vi "Main_ch.vi"() -> ()   [LabVIEW 2020]
uses:
  <vilib>/Utility/error.llb/DialogType.ctl
  <vilib>/DAQmx/read.llb/DAQmx Read (Analog 1D Wfm NChan NSamp).vi
  <extravilib>/ChannelInstances/Tag-bool/Read With Abort.vi
  <extravilib>/ChannelInstances/Tag-bool/Write With Abort.vi
  <vilib>/ULx/Create Channel.llb/ULx Create Channel (AI-Voltage-Basic).vi
  <vilib>/ULx/Timing.llb/ULx Timing (Sample Clock).vi
  <vilib>/DAQmx/create/channels.llb/DAQmx Create Channel (AI-Acceleration-Accelerometer).vi
  <vilib>/DAQmx/configure/timing.llb/DAQmx Timing (Sample Clock).vi
  <vilib>/DAQmx/configure/trigger.llb/DAQmx Start Trigger (Digital Edge).vi
  <vilib>/DAQmx/configure/trigger.llb/DAQmx Start Trigger (Time).vi
  <vilib>/DAQmx/configure/trigger.llb/DAQmx Start Trigger (Analog Edge).vi
  <extravilib>/ChannelInstances/Tag-bool/Instantiate.vi
  <extravilib>/ChannelInstances/Tag-bool/EndpointRead.vi
  <vilib>/ULx/Read.llb/ULx Read (Analog Wfm 1Chan NSamp).vi
  <vilib>/Waveform/DWDTOps.llb/DWDT Digital to Binary U16.vi
  <vilib>/ULx/Read.llb/ULx Read (Analog 1D Wfm NChan NSamp).vi
  <vilib>/DAQmx/miscellaneous.llb/DAQmx Fill In Error Info.vi
  <extravilib>/ChannelInstances/Tag-bool/Endpoint.vi
  <extravilib>/ChannelInstances/Tag-bool.lvlib
  <resource>/objmgr/daqmx.rc
panel:
  out "Power Graph":waveform(dbl)(graph)
  out "Tach Graph":digitalwaveform[](graph)
  out "Torque Graph":waveform(dbl)(graph)
  in  "Trigger Type":T1(tab)
  in  "Digital Start Trigger Edge":i32(ring)=10280 caption="Edge" items=["Rising"=10280, "Falling"=10171]
  in  "Digital Start Trigger Source":tag="/Dev1/PFI0" caption="Source"
  in  "Digital Pause Trigger Pause When":i32(ring)=10192 caption="Pause When" items=["High"=10192, "Low"=10214]
  in  "Digital Pause Trigger Source":tag="/Dev1/PFI0" caption="Source"
  in  "Analog Start Trigger Level":dbl caption="Level" format="%0.2f"
  in  "Analog Start Trigger Hysteresis":dbl caption="Hysteresis" format="%.2f"
  in  "Analog Start Trigger Slope":i32(ring)=10280 caption="Slope" items=["Rising"=10280, "Falling"=10171]
  in  "Analog Start Trigger Source":string="APFI0" caption="Source"
  in  "Analog Pause Trigger Source":string="APFI0" caption="Source"
  in  "Analog Pause Trigger Pause When":i32(ring)=10093 caption="Pause When" items=["Above Level"=10093, "Below Level"=10107]
  in  "Analog Pause Trigger Level":dbl caption="Level" format="%.2f"
  in  "When":timestamp
  in  "Select Time\nManually":bool
  out "Accel Graph":waveform(dbl)[](graph)
  out "Actual Sample Rate":dbl=1000.0 format="%0.2f"
  out "Mic Graph":dynamicdata(graph)
  out "Load Cell Graph":waveform(dbl)[](graph)
  in  "stop":bool
  # "To enable triggers, select a tab above, and configure the settings.\n\nNot all hardware supports all trigger types. Refer to your device documentation for more information."
  # "This trigger type is not supported in continuous sample timing. \n\nRefer to your device documentation for more information on which triggers are supported."
  # "This trigger type is not supported in continuous sample timing. \n\nRefer to your device documentation for more information on which triggers are supported."
  # "If time is not manually set, task will begin after 10 seconds"
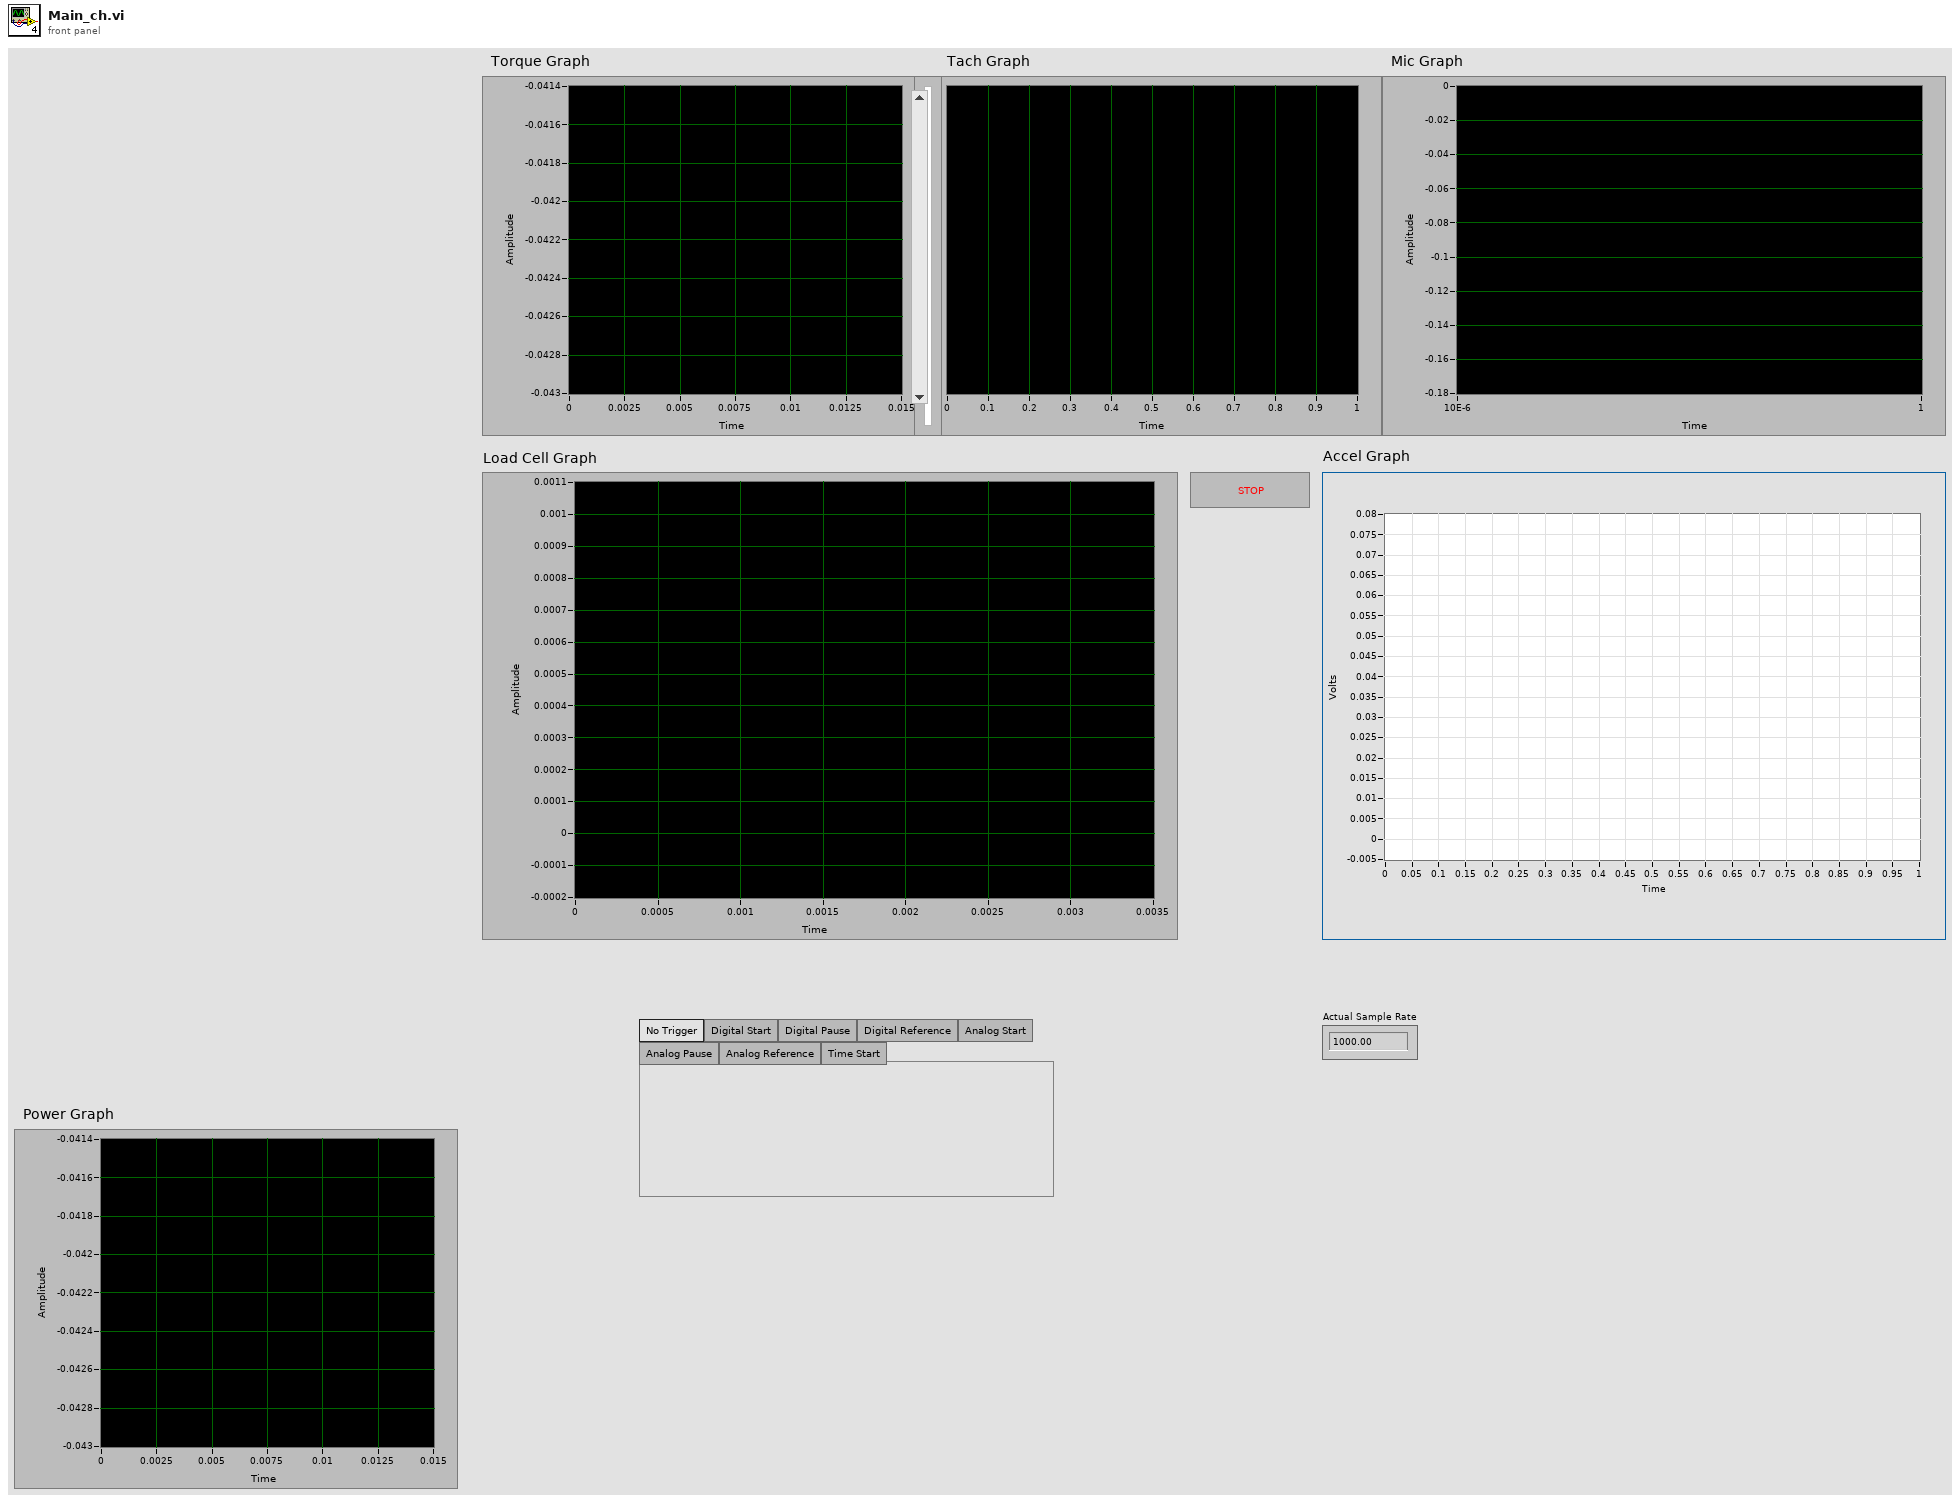
[diagram p1: front panel]
types:
  T1 = enum32{"No Trigger", "Digital Start", "Digital Pause", "Digital Reference", "Analog Start", "Analog Pause", "Analog Reference", "Time Start"}
  T2 = typedef "DialogType.ctl" = u16
  T3 = typedef "Tag-bool.lvlib/))Channel.ctl" = refnum<queue>
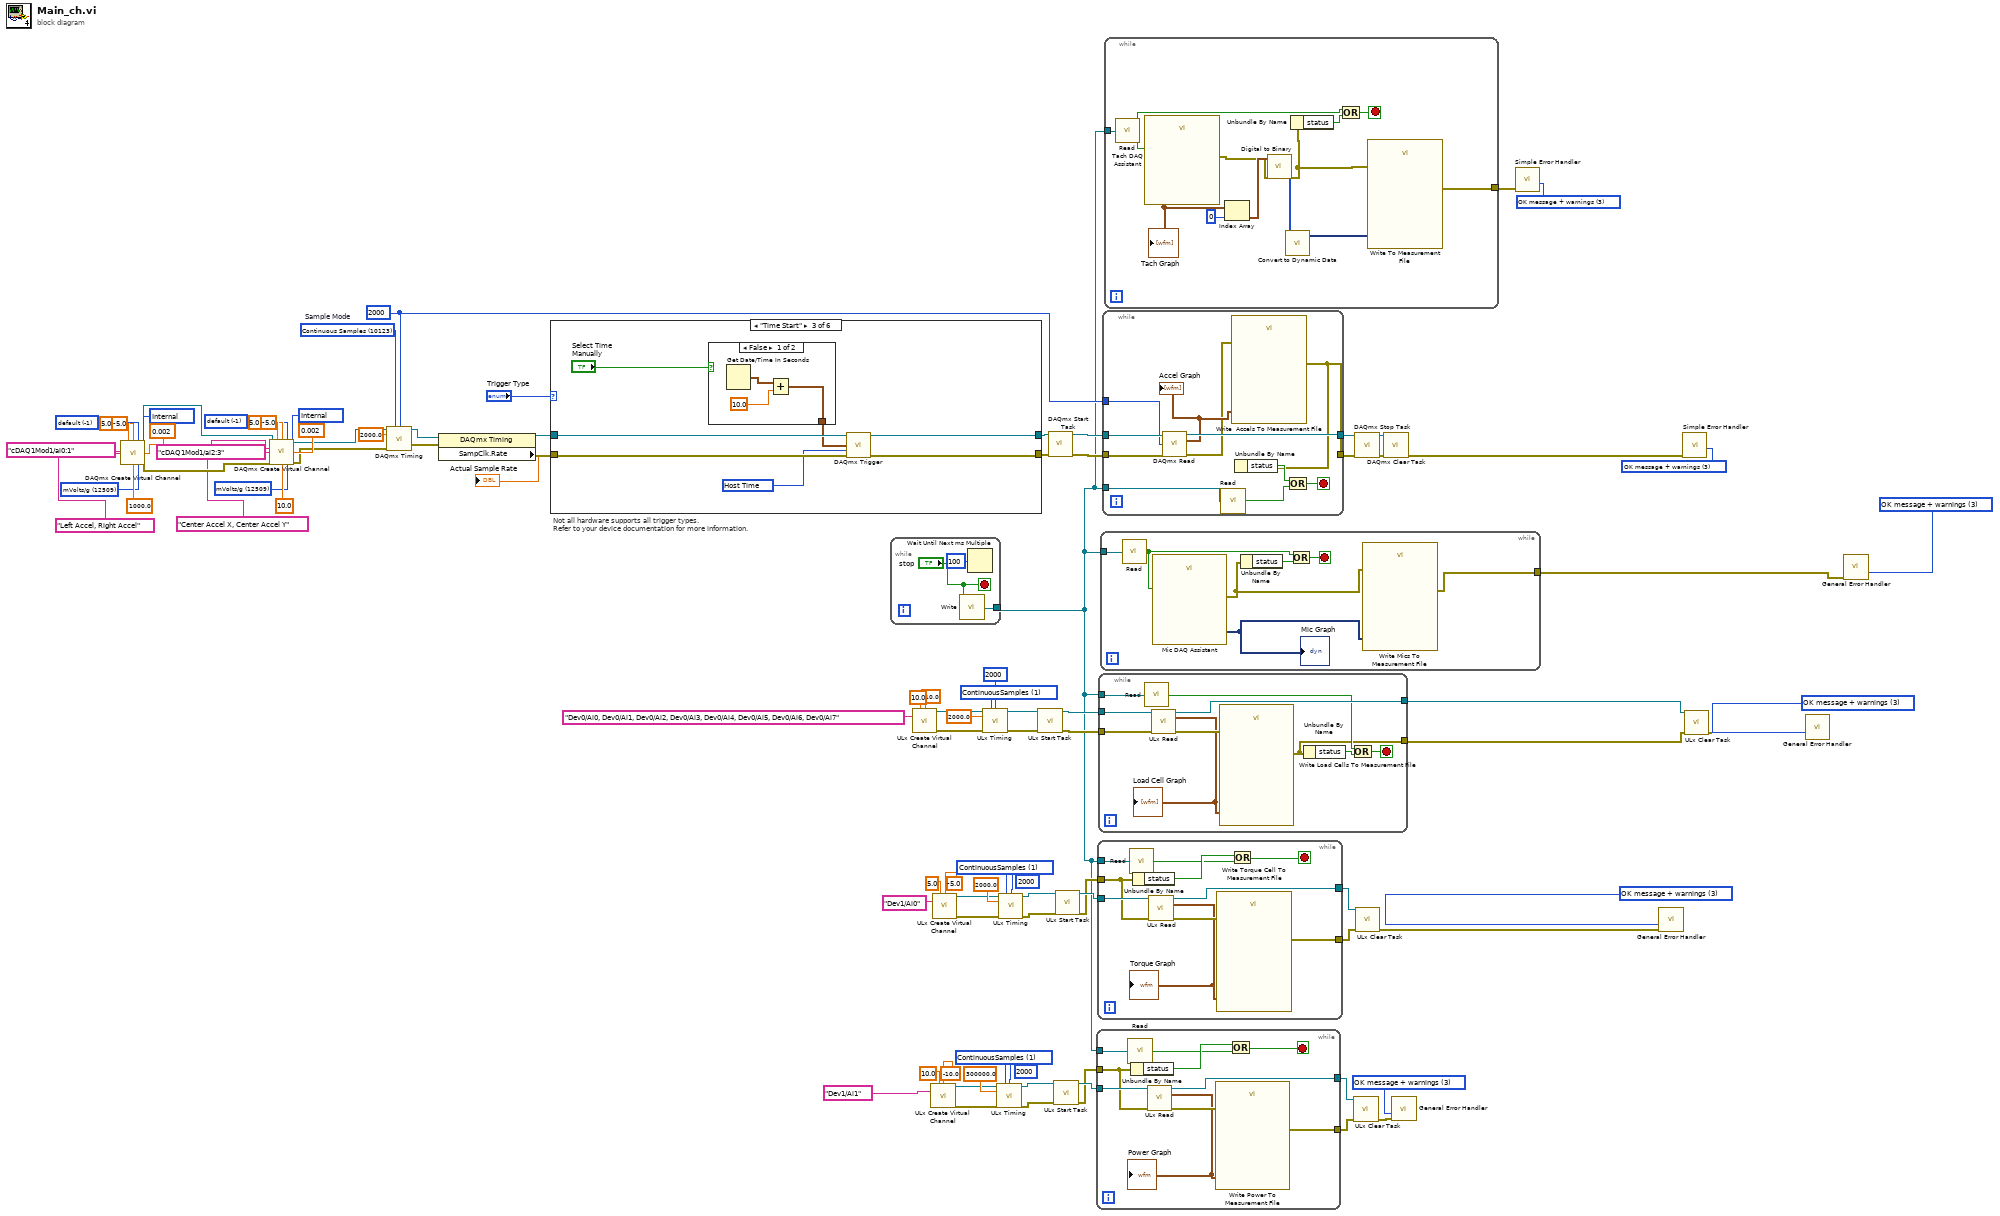
[diagram p0: block diagram]
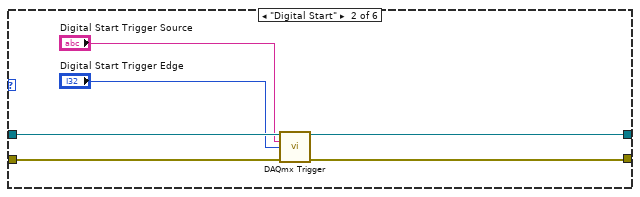
[diagram p3: hidden frame]
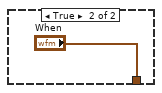
[diagram p4: hidden frame]
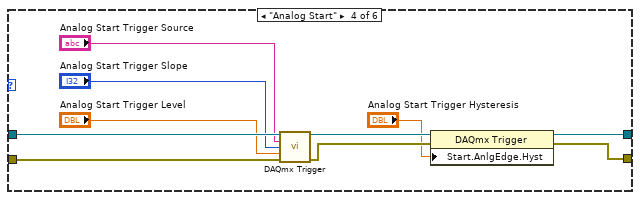
[diagram p5: hidden frame]
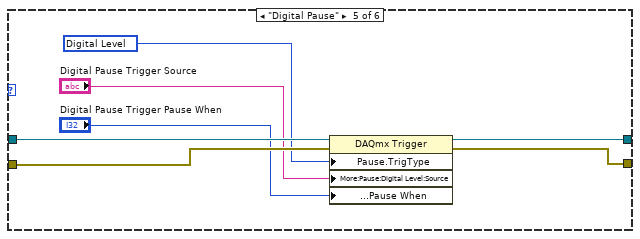
[diagram p6: hidden frame]
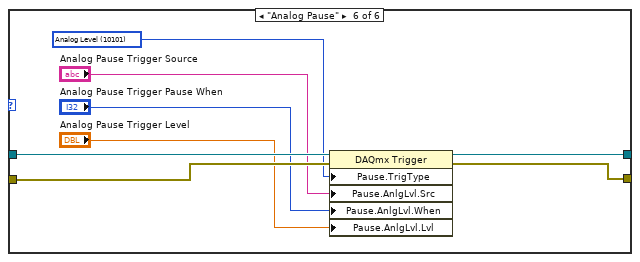
[diagram p7: hidden frame]
diagram:
  w14 = 1 items=["FiniteSamples", "ContinuousSamples"] ("sample mode")
  w11 = T2 3 items=["no dialog", "OK message", "continue or stop message", "OK message + warnings", "continue/stop + warnings"] ("type of dialog (OK msg:1)")
  w20 = T2 3 items=["no dialog", "OK message", "continue or stop message", "OK message + warnings", "continue/stop + warnings"] ("type of dialog (OK msg:1)")
  w35 = 1 items=["FiniteSamples", "ContinuousSamples"] ("sample mode")
  w32 = T2 3 items=["no dialog", "OK message", "continue or stop message", "OK message + warnings", "continue/stop + warnings"] ("type of dialog (OK msg:1)")
  w47 = 12509 items=["mVolts/g"=12509, "Volts/g"=12510] ("sensitivity units")
  w48 = 12509 items=["mVolts/g"=12509, "Volts/g"=12510] ("sensitivity units")
  w52 = 10200 items=["Internal"=10200, "External"=10167, "None"=10230] ("current excitation source")
  w53 = -1 items=["default"=-1, "RSE"=10083, "NRSE"=10078, "Differential"=10106, "Pseudodifferential"=12529] ("input terminal configuration")
  w57 = 2000 ("samples per channel")
  w62 = T2 3 items=["no dialog", "OK message", "continue or stop message", "OK message + warnings", "continue/stop + warnings"] ("type of dialog (OK msg:1)")
  w73 = 10123 items=["Finite Samples"=10178, "Continuous Samples"=10123, "Hardware Timed Single Point"=12522]  # Sample Mode
  w77 = 10200 items=["Internal"=10200, "External"=10167, "None"=10230] ("current excitation source")
  w78 = -1 items=["default"=-1, "RSE"=10083, "NRSE"=10078, "Differential"=10106, "Pseudodifferential"=12529] ("input terminal configuration")
  w82 = T2 3 items=["no dialog", "OK message", "continue or stop message", "OK message + warnings", "continue/stop + warnings"] ("type of dialog (OK msg:1)")
  w86 = 1 items=["FiniteSamples", "ContinuousSamples"] ("sample mode")
  w90 = T2 3 items=["no dialog", "OK message", "continue or stop message", "OK message + warnings", "continue/stop + warnings"] ("type of dialog (OK msg:1)")
  # "Not all hardware supports all trigger types.\nRefer to your device documentation for more information."
  n1 = call-poly <vilib>:"DAQmx Create Virtual Channel.vi"("maximum value"=5.0, "minimum value"=-5.0, "input terminal configuration"=w78, "physical channels"=tag "cDAQ1Mod1/ai0:1", "current excitation source"=w77, "name to assign"="Left Accel, Right Accel", "current excitation value"=0.002, "sensitivity"=1000.0, "sensitivity units"=w47) -> ("task out"=w44:refnum<k21>, "error out"=w45:errorcluster)  [unwired: 5 in]
  n2 = call-poly <vilib>:"DAQmx Create Virtual Channel.vi"("task in"=w44, "maximum value"=5.0, "minimum value"=-5.0, "input terminal configuration"=w53, "physical channels"=tag "cDAQ1Mod1/ai2:3", "current excitation source"=w52, "name to assign"="Center Accel X, Center Accel Y", "current excitation value"=0.002, "error in"=w45, "sensitivity"=10.0, "sensitivity units"=w48) -> ("task out"=w43:refnum<k21>, "error out"=w46:errorcluster)  [unwired: 3 in]
  n3 = call-poly <vilib>:"DAQmx Timing.vi"("task/channels in"=w43, "sample mode"=w73, "samples per channel"=w57, "rate"=2000.0, "error in"=w46) -> ("task out"=w75:refnum<k21>, "error out"=w74:errorcluster)  [unwired: 9 in]
  n4 = property class="DAQmx Timing"(reference=w75, error in=w74) -> (reference out=w72:refnum<k21>, error out=w71:errorcluster, "SampClk.Rate"=→"Actual Sample Rate":dbl)
  n5 = case shown="\"Time Start\"" "Trigger Type" {
    tunnel: w72 -> [w96 w102 w109 w123 w130 w138]
    tunnel: w71 -> [w95 w101 w108 w122 w127 w135]
    tunnel: [w96 w100 w107 w120 w129 w137] -> w59
    tunnel: [w95 w99 w106 w119 w128 w136] -> w60
    frame "No Trigger", Default {
    }
    frame "Digital Start" {
      n6 = call-poly <vilib>:"DAQmx Trigger.vi"("task/channels in"=w102, "source"="Digital Start Trigger Source", "edge"="Digital Start Trigger Edge", "error in"=w101) -> ("task out"=w100:refnum<k21>, "error out"=w99:errorcluster)  [unwired: 10 in]
    }
    frame "Time Start" {
      w105 = 16126 items=["Host Time"=16126, "I/O Device Time"=16127] ("timescale")
      n7 = case shown="False" "Select Time\nManually" {
        tunnel: [w110 "When"] -> w103
        frame False {
          n8 = Get Date/Time In Seconds() -> (seconds since 1Jan1904=w112:timestamp)
          n9 = Add(x=w112, y=10.0) -> (x+y=w110:timestamp)
        }
        frame True {
        }
      }
      n10 = call-poly <vilib>:"DAQmx Trigger.vi"("task/channels in"=w109, "when"=w103, "timescale"=w105, "error in"=w108) -> ("task out"=w107:refnum<k21>, "error out"=w106:errorcluster)  [unwired: 10 in]
    }
    frame "Analog Start" {
      n11 = call-poly <vilib>:"DAQmx Trigger.vi"("task/channels in"=w123, "source"="Analog Start Trigger Source", "slope"="Analog Start Trigger Slope", "level"="Analog Start Trigger Level", "error in"=w122) -> ("task out"=w118:refnum<k21>, "error out"=w117:errorcluster)  [unwired: 9 in]
      n12 = property class="DAQmx Trigger"(reference=w118, error in=w117, "Start.AnlgEdge.Hyst"="Analog Start Trigger Hysteresis") -> (reference out=w120:refnum<k21>, error out=w119:errorcluster)
    }
    frame "Digital Pause" {
      w126 = 10152 items=["Analog Level"=10101, "Analog Window"=10103, "Digital Level"=10152, "Digital Pattern"=10398, "None"=10230] ("Pause.TrigType")
      n13 = property class="DAQmx Trigger"(reference=w130, error in=w127, "Pause.TrigType"=w126, "More:Pause:Digital Level:Source"="Digital Pause Trigger Source", "More:Pause:Digital Level:Pause When"="Digital Pause Trigger Pause When") -> (reference out=w129:refnum<k21>, error out=w128:errorcluster)
    }
    frame "Analog Pause" {
      w134 = 10101 items=["Analog Level"=10101, "Analog Window"=10103, "Digital Level"=10152, "Digital Pattern"=10398, "None"=10230] ("Pause.TrigType")
      n14 = property class="DAQmx Trigger"(reference=w138, error in=w135, "Pause.TrigType"=w134, "Pause.AnlgLvl.Src"="Analog Pause Trigger Source", "Pause.AnlgLvl.When"="Analog Pause Trigger Pause When", "Pause.AnlgLvl.Lvl"="Analog Pause Trigger Level") -> (reference out=w137:refnum<k21>, error out=w136:errorcluster)
    }
  }
  n15 = while {
    tunnel: [w139] -> w2
    stop <- "stop" stop-if-true
    n16 = call <extravilib>:"Write.vi"("element"="stop") -> ("channel"=w139:T3)  [unwired: 1 out]
    n17 = Wait Until Next ms Multiple(millisecond multiple=u32 100 ("millisecond timer value")) -> ()  [unwired: 1 out]
  }
  n18 = call-poly <vilib>:"ULx Create Virtual Channel.vi"("maximum value"=10.0, "minimum value"=-10.0, "physical channels"="Dev0/Ai0, Dev0/Ai1, Dev0/Ai2, Dev0/Ai3, Dev0/Ai4, Dev0/Ai5, Dev0/Ai6, Dev0/Ai7") -> ("task out"=w92:refnum<k24>, "error out"=w94:errorcluster)  [unwired: 11 in]
  n19 = call-poly <vilib>:"ULx Create Virtual Channel.vi"("maximum value"=10.0, "minimum value"=-10.0, "physical channels"="Dev1/Ai1") -> ("task out"=w7:refnum<k24>, "error out"=w4:errorcluster)  [unwired: 11 in]
  n20 = call-poly <vilib>:"ULx Create Virtual Channel.vi"("maximum value"=5.0, "minimum value"=-5.0, "physical channels"="Dev1/Ai0") -> ("task out"=w28:refnum<k24>, "error out"=w25:errorcluster)  [unwired: 11 in]
  n21 = call-poly <vilib>:"ULx Timing.vi"("task in"=w92, "sample mode"=w86, "samples per channel"=2000, "rate"=2000.0, "error in"=w94) -> ("task out"=w42:refnum<k24>, "error out"=w89:errorcluster)  [unwired: 9 in]
  n22 = call-poly <vilib>:"ULx Timing.vi"("task in"=w7, "sample mode"=w14, "samples per channel"=2000, "rate"=300000.0, "error in"=w4) -> ("task out"=w12:refnum<k24>, "error out"=w13:errorcluster)  [unwired: 9 in]
  n23 = call-poly <vilib>:"ULx Timing.vi"("task in"=w28, "sample mode"=w35, "samples per channel"=2000, "rate"=2000.0, "error in"=w25) -> ("task out"=w33:refnum<k24>, "error out"=w34:errorcluster)  [unwired: 9 in]
  n24 = call <vilib>:"ULx Start Task.vi"("task in"=w42, "error in"=w89) -> ("task out"=w91:refnum<k24>, "error out"=w93:errorcluster)  [unwired: 12 in]
  n25 = call <vilib>:"DAQmx Start Task.vi"("task/channels in"=w59, "error in"=w60) -> ("task out"=w70:refnum<k21>, "error out"=w69:errorcluster)  [unwired: 12 in]
  n26 = call <vilib>:"ULx Start Task.vi"("task in"=w12, "error in"=w13) -> ("task out"=w8:refnum<k24>, "error out"=w5:errorcluster)  [unwired: 12 in]
  n27 = call <vilib>:"ULx Start Task.vi"("task in"=w33, "error in"=w34) -> ("task out"=w29:refnum<k24>, "error out"=w26:errorcluster)  [unwired: 12 in]
  n28 = while {
    tunnel: w5 -> [w145]
    tunnel: w8 -> [w151]
    tunnel: [w150] -> w9
    tunnel: [w146] -> w10
    tunnel: w2 -> [w144]
    stop <- w148 stop-if-true
    n29 = call <extravilib>:"Read.vi"("channel"=w144) -> ("element"=w143:bool)  [unwired: 1 in, 1 out]
    n30 = Unbundle By Name(w145) -> ("status"=w149:bool)
    n31 = call-poly <vilib>:"ULx Read.vi"("task in"=w151, "error in"=w145) -> ("task out"=w150:refnum<k24>, "data"=w142:waveform(dbl), "error out"=w147:errorcluster)  [unwired: 11 in]
    "Power Graph" <- w142
    n32 = call "Write Power To Measurement File"("Signals"=w142, "error in (no error)"=w147) -> ("error out"=w146:errorcluster)  [unwired: 15 in, 2 out]
    n33 = Or(x=w149, y=w143) -> (x .or. y?=w148:bool)
  }
  n34 = while {
    tunnel: w26 -> [w155]
    tunnel: w29 -> [w161]
    tunnel: [w160] -> w30
    tunnel: [w156] -> w31
    tunnel: w2 -> [w154]
    stop <- w158 stop-if-true
    n35 = call <extravilib>:"Read.vi"("channel"=w154) -> ("element"=w153:bool)  [unwired: 1 in, 1 out]
    n36 = Unbundle By Name(w155) -> ("status"=w159:bool)
    n37 = call-poly <vilib>:"ULx Read.vi"("task in"=w161, "error in"=w155) -> ("task out"=w160:refnum<k24>, "data"=w152:waveform(dbl), "error out"=w157:errorcluster)  [unwired: 11 in]
    "Torque Graph" <- w152
    n38 = call "Write Torque Cell To Measurement File"("Signals"=w152, "error in (no error)"=w157) -> ("error out"=w156:errorcluster)  [unwired: 15 in, 2 out]
    n39 = Or(x=w159, y=w153) -> (x .or. y?=w158:bool)
  }
  n40 = while {
    tunnel: w93 -> [w168]
    tunnel: w91 -> [w171]
    tunnel: [w170] -> w23
    tunnel: w2 -> [w167]
    tunnel: [w163] -> w22
    stop <- w169 stop-if-true
    n41 = call <extravilib>:"Read.vi"("channel"=w167) -> ("element"=w165:bool)  [unwired: 1 in, 1 out]
    n42 = call-poly <vilib>:"ULx Read.vi"("task in"=w171, "error in"=w168) -> ("task out"=w170:refnum<k24>, "data"=w162:waveform(dbl)[], "error out"=w164:errorcluster)  [unwired: 11 in]
    "Load Cell Graph" <- w162
    n43 = call "Write Load Cells To Measurement File"("Signals"=w162, "error in (no error)"=w164) -> ("error out"=w163:errorcluster)  [unwired: 15 in, 2 out]
    n44 = Unbundle By Name(w163) -> ("status"=w166:bool)
    n45 = Or(x=w165, y=w166) -> (x .or. y?=w169:bool)
  }
  n46 = while {
    tunnel: w2 -> [w178]
    tunnel: [w174] -> w19
    stop <- w177 stop-if-true
    n47 = call <extravilib>:"Read.vi"("channel"=w178) -> ("element"=w176:bool)  [unwired: 1 in, 1 out]
    n48 = call "Mic DAQ Assistant"("stop (F)"=w176) -> ("data"=w173:dynamicdata, "error out"=w172:errorcluster)  [unwired: 15 in, 2 out]
    "Mic Graph" <- w173
    n49 = Unbundle By Name(w172) -> ("status"=w175:bool)
    n50 = Or(x=w176, y=w175) -> (x .or. y?=w177:bool)
    n51 = call "Write Mics To Measurement File"("Signals"=w173, "error in (no error)"=w172) -> ("error out"=w174:errorcluster)  [unwired: 15 in, 2 out]
  }
  n52 = while {
    tunnel: w70 -> [w189]
    tunnel: w69 -> [w188]
    tunnel: [w187] -> w66
    tunnel: [w179] -> w65
    tunnel: w57 -> [w184]
    tunnel: w2 -> [w182]
    stop <- w185 stop-if-true
    n53 = call-poly <vilib>:"DAQmx Read.vi"("task/channels in"=w189, "number of samples per channel"=w184, "error in"=w188) -> ("task out"=w187:refnum<k21>, "data"=w181:waveform(dbl)[], "error out"=w180:errorcluster)  [unwired: 10 in]
    "Accel Graph" <- w181
    n54 = call <extravilib>:"Read.vi"("channel"=w182) -> ("element"=w183:bool)  [unwired: 1 in, 1 out]
    n55 = call "Write  Accels To Measurement File"("Signals"=w181, "error in (no error)"=w180) -> ("error out"=w179:errorcluster)  [unwired: 15 in, 2 out]
    n56 = Unbundle By Name(w179) -> ("status"=w186:bool)
    n57 = Or(x=w186, y=w183) -> (x .or. y?=w185:bool)
  }
  n58 = while {
    tunnel: w2 -> [w201]
    tunnel: [w197] -> w1
    stop <- w200 stop-if-true
    n59 = call <extravilib>:"Read.vi"("channel"=w201) -> ("element"=w198:bool)  [unwired: 1 in, 1 out]
    n60 = call "Tach DAQ Assistant"("stop (F)"=w198) -> ("data"=w194:digitalwaveform[], "error out"=w191:errorcluster)  [unwired: 15 in, 2 out]
    "Tach Graph" <- w194
    n61 = Index Array(array=w194, index=0) -> (element=w192:digitalwaveform)
    n62 = call-poly <vilib>:"Digital to Binary.vi"("error in (no error)"=w191, "digital waveform"=w192) -> ("error out"=w190:errorcluster, "binary array"=w196:u16[])  [unwired: 8 in]
    n63 = call "Convert to Dynamic Data"("Array"=w196) -> ("Dynamic Data Type"=w195:dynamicdata)  [unwired: 3 in]
    n64 = Unbundle By Name(w190) -> ("status"=w199:bool)
    n65 = Or(x=w198, y=w199) -> (x .or. y?=w200:bool)
    n66 = call "Write To Measurement File"("Signals"=w195, "error in (no error)"=w190) -> ("error out"=w197:errorcluster)  [unwired: 15 in, 2 out]
  }
  n67 = call <vilib>:"ULx Clear Task.vi"("task in"=w9, "error in"=w10) -> ("error out"=w6:errorcluster)  [unwired: 13 in]
  n68 = call <vilib>:"DAQmx Stop Task.vi"("task/channels in"=w66, "error in"=w65) -> ("task out"=w63:refnum<k21>, "error out"=w64:errorcluster)  [unwired: 12 in]
  n69 = call <vilib>:"ULx Clear Task.vi"("task in"=w30, "error in"=w31) -> ("error out"=w27:errorcluster)  [unwired: 13 in]
  n70 = call <vilib>:"DAQmx Clear Task.vi"("task in"=w63, "error in"=w64) -> ("error out"=w68:errorcluster)  [unwired: 13 in]
  n71 = call <vilib>:"General Error Handler.vi"("type of dialog (OK msg:1)"=w11, "error in (no error)"=w6) -> ()  [unwired: 9 in, 5 out]
  n72 = call <vilib>:"Simple Error Handler.vi"("type of dialog (OK msg:1)"=w20, "error in (no error)"=w1) -> ()  [unwired: 3 in, 5 out]
  n73 = call <vilib>:"General Error Handler.vi"("type of dialog (OK msg:1)"=w32, "error in (no error)"=w27) -> ()  [unwired: 9 in, 5 out]
  n74 = call <vilib>:"Simple Error Handler.vi"("type of dialog (OK msg:1)"=w62, "error in (no error)"=w68) -> ()  [unwired: 3 in, 5 out]
  n75 = call <vilib>:"ULx Clear Task.vi"("task in"=w23, "error in"=w22) -> ("error out"=w21:errorcluster)  [unwired: 13 in]
  n76 = call <vilib>:"General Error Handler.vi"("type of dialog (OK msg:1)"=w90, "error in (no error)"=w21) -> ()  [unwired: 9 in, 5 out]
  n77 = call <vilib>:"General Error Handler.vi"("type of dialog (OK msg:1)"=w82, "error in (no error)"=w19) -> ()  [unwired: 9 in, 5 out]
